vi "Start Create.vi"(6 "Alias":string, 9 "Actor":refnum<class "Actor.lvclass">, 10 "Actor in":refnum<class "Actor.lvclass">) -> (0 "Error out":errorcluster, 2 "Actor out":refnum<class "Actor.lvclass">)   [LabVIEW 2020, in "jettl.lvlib" / "Actor.lvlib"]
uses:
  Actor.lvlib
  Actor/Actor.lvclass
  Error/Error.lvlib
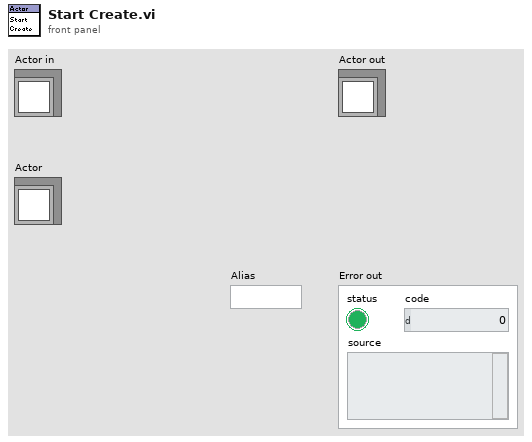
[diagram p1: front panel]
types:
  T1 = typedef "jettl.lvlib/Actor.lvlib/Created Aliases.ctl" = set{string}
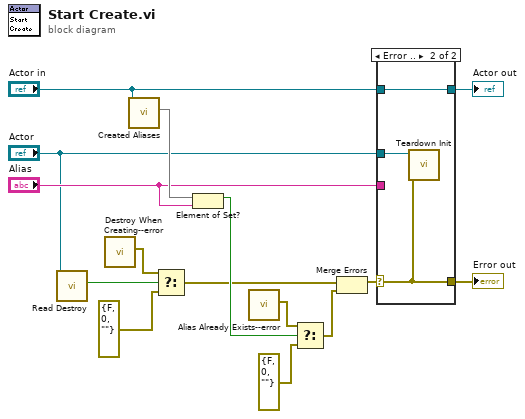
[diagram p0: block diagram]
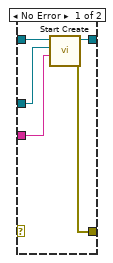
[diagram p2: hidden frame]
diagram:
  n1 = call-dynamic "Read Destroy.vi"("Actor in"="Actor") -> ("Destroy"=w7:bool)  [unwired: 10 in]
  n2 = call "Destroy When Creating--error.vi"() -> ("Error"=w8:errorcluster)  [unwired: 11 in]
  n3 = call-dynamic "Created Aliases.vi"("Actor in"="Actor in") -> ("Created Aliases"=w13:T1)  [unwired: 10 in]
  n4 = Select(t=w8, s=w7, f=errorcluster {"status"=FALSE, "code"=0, "source"=""}) -> (s? t:f=w1:errorcluster)
  n5 = Element of Set?(10:"Alias", 11:w13) -> (3:w4:bool)
  n6 = call "Alias Already Exists--error.vi"() -> ("Error"=w5:errorcluster)  [unwired: 11 in]
  n7 = Select(t=w5, s=w4, f=errorcluster {"status"=FALSE, "code"=0, "source"=""}) -> (s? t:f=w2:errorcluster)
  n8 = Merge Errors(w1, w2) -> (w10:errorcluster)
  n9 = case shown="Error .." w10 {
    selector: w10 -> [_ w21]
    tunnel: "Alias" -> [w16 _]
    tunnel: "Actor in" -> [w18 w23]
    tunnel: [w20 w21] -> w15
    tunnel: [w19 w23] -> w14
    tunnel: "Actor" -> [w17 w22]
    frame No Error {
      n10 = call-dynamic "Start Create.vi"("Alias"=w16, "Actor"=w17, "Actor in"=w18) -> ("Error out"=w20:errorcluster, "Actor out"=w19:refnum<class "Actor.lvclass">)  [unwired: 7 in]
    }
    frame Error {
      n11 = call-dynamic "Teardown Init.vi"("Error in"=w21, "Actor in"=w22) -> ()  [unwired: 9 in, 1 out]
    }
  }
  "Error out" <- w15
  "Actor out" <- w14
